vi "Slice Engine.vi"(7 "Table Stages":T3={"X Stage"={"Position"=0.0, "Is.Enabled?"=FALSE, "Is.Connected?"=FALSE, "Device SN"="45876425", "AccelerationMaximum"=20.0, "VelocityMaximum"=20.0, "Acceleration"=15.0, "Velocity"=18.0, "waitTimeout (ms)"=500000, "Model"=enum."None", "Is.Homed?"=FALSE, "MOVE"=FALSE}, "Y Stage"={"Position"=0.0, "Is.Enabled?"=FALSE, "Is.Connected?"=FALSE, "Device SN"="45995820", "AccelerationMaximum"=20.0, "VelocityMaximum"=20.0, "Acceleration"=15.0, "Velocity"=18.0, "waitTimeout (ms)"=5000000, "Model"=enum."None", "Is.Homed?"=FALSE, "MOVE"=FALSE}, "Z Stage"={"Position"=0.0, "Is.Enabled?"=FALSE, "Is.Connected?"=FALSE, "Device SN"="49103464", "AccelerationMaximum"=0.0, "VelocityMaximum"=0.0, "Acceleration"=0.0, "Velocity"=0.0, "waitTimeout (ms)"=0, "Model"=enum."None", "Is.Homed?"=FALSE, "MOVE"=FALSE}}, 8 "error in (no error)":errorcluster, 9 "Vibratome":T1={"Z Bottom [mm]"=0.0, "Pre Cut Dwell [s]"=0.0, "Blade Frequency [RPM]"=0, "Slice Speed [mm/s]"=0.0, "Post Cut Dwell [s]"=0.0, "Ramp Time [s]"=0.0, "Start X [mm]"=0.0, "Start Y [mm]"=0.0, "Slice Length [mm]"=0.0, "Slice Axis"=enum."X Axis", "Controller VISA Ref"="COM4", "Blade Frequency [Hz]"=0, "Analog Out Channel"="GalvoCtrl/ao0,GalvoCtrl/ao1", "Pixel Clock Source"="/GalvoCtrl/PFI0", "Vib"=enum."Vibratome1"}, 10 "Action":string="Init", 11 "Last Slice?":bool) -> (0 "error out":errorcluster)   [LabVIEW 2018]
uses:
  Controls/Translation Stage Parameters.ctl
  Hardware Mfg/Thorlabs Translation Stages/Controls/Translation Stage Cluster.ctl
  Controls/Translation Stage Types.ctl
  Controls/Vibratome Parameters.ctl
  type defines/vibratome.ctl
  Controls/Queue Manager Actions.ctl
  Controls/QueueNames.ctl
  Controls/Set Get Controls.ctl
  Hardware Mfg/Thorlabs Translation Stages/Controls/Motion Translation Module Control2.ctl
  Hardware Mfg/Thorlabs Translation Stages/Controls/Motion Translation Module Control.ctl
  Controls/vibratome3 control.ctl
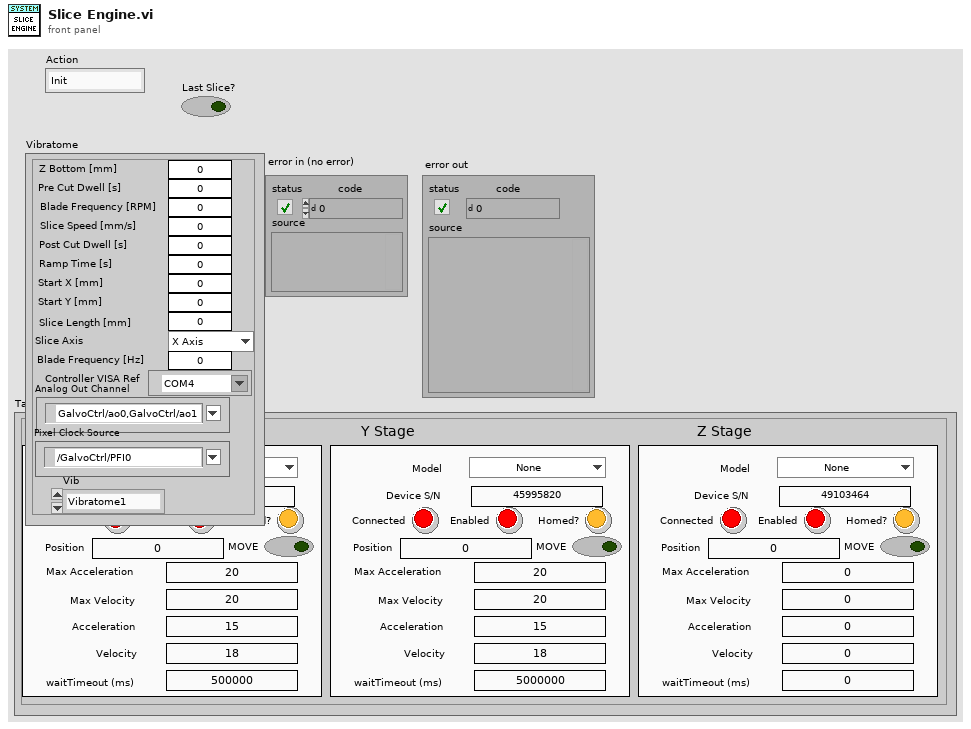
[diagram p1: front panel]
types:
  T1 = typedef "Vibratome Parameters.ctl" = cluster{"Z Bottom [mm]":dbl, "Pre Cut Dwell [s]":dbl, "Blade Frequency [RPM]":u16, "Slice Speed [mm/s]":dbl, "Post Cut Dwell [s]":dbl, "Ramp Time [s]":dbl, "Start X [mm]":dbl, "Start Y [mm]":dbl, "Slice Length [mm]":dbl, "Slice Axis":enum16{"X Axis", "Y Axis", "Z Axis"}, "Controller VISA Ref":refnum<visa-resource-name>, "Blade Frequency [Hz]":u16, "Analog Out Channel":tag, "Pixel Clock Source":tag, "Vib":T2}
  T2 = typedef "vibratome.ctl" = enum16{"Vibratome1", "Vibratome3"}
  T3 = typedef "Translation Stage Parameters.ctl" = cluster{"X Stage":T4, "Y Stage":T4, "Z Stage":T4}
  T4 = typedef "Translation Stage Cluster.ctl" = cluster{"Position":dbl, "Is.Enabled?":bool, "Is.Connected?":bool, "Device SN":string, "AccelerationMaximum":dbl, "VelocityMaximum":dbl, "Acceleration":dbl, "Velocity":dbl, "waitTimeout (ms)":i32, "Model":T5, "Is.Homed?":bool, "MOVE":bool}
  T5 = typedef "Translation Stage Types.ctl" = enum16{"None", "Thorlabs LTS", "Thorlabs MLJ"}
  T6 = typedef "QueueNames.ctl" = enum16{"Main GUI", "Main Scan Processor", "Main Processing", "Main Saving", "Main Display", "Main Table Stage GUI", "Main Table Stage Proc.", "Scan Engine", "Vibratome GUI", "Vibratome Processor", "Slice Engine"}
  T7 = typedef "Queue Manager Actions.ctl" = enum16{"Init", "Enqueue", "Enqueue All", "Preview Queue", "Dequeue", "Get Status", "Flush Queue", "Flush All Queues", "Release All Queues", "Release Queue", "Enqueue at Opposite End"}
  T8 = typedef "Set Get Controls.ctl" = enum16{"Set", "Get"}
  T9 = typedef "Motion Translation Module Control.ctl" = enum16{"Init", "Home", "Status", "Velocity/Accel", "Position", "Jog", "Stop", "Uninit", "Enable", "Disable"}
  T10 = typedef "Motion Translation Module Control2.ctl" = enum16{"Init", "Home", "Status", "Velocity/Accel", "Position", "Jog", "Stop", "Uninit", "Enable", "Disable"}
  T11 = enum16{"Set Configuration", "Get Configuration", "Enable Motor", "Disable Motor", "Get Status", "Open Session", "Close Session", "Set Limits", "Get Limits"}
  T12 = cluster{"Source for Velocity":enum16{"Interface", "Voltage (AI)", "PWM (AI)", "Current Target (AI)", "Current Target w/ Preset (AI)"}, "Mode":enum16{"Continuous", "Stepper Motor", "Analog Position Ctrl", "Encoder"}, "Target Velocity [RPM]":i16}
  T13 = typedef "vibratome3 control.ctl" = enum16{"Init", "Configure channel", "Write waveform", "Start", "Stop", "Finish?", "Uninit"}
  T14 = typedef "Motion Translation Module Control.ctl" = enum16{"Uninit", "Measure power", "Move angle", "Gen angles", "Init cage", "Init PM"}
  T15 = typedef "MessagePacket.ctl" = cluster{"Message":string, "Parameter":variant}
  T16 = typedef "Translation Stage Quick Status.ctl" = cluster{"Is.Enabled?":bool, "Is.Connected?":bool, "Is.Homed?":bool}
  T17 = enum16{"Left Button", "Center Button", "Right Button", "Window Close"}
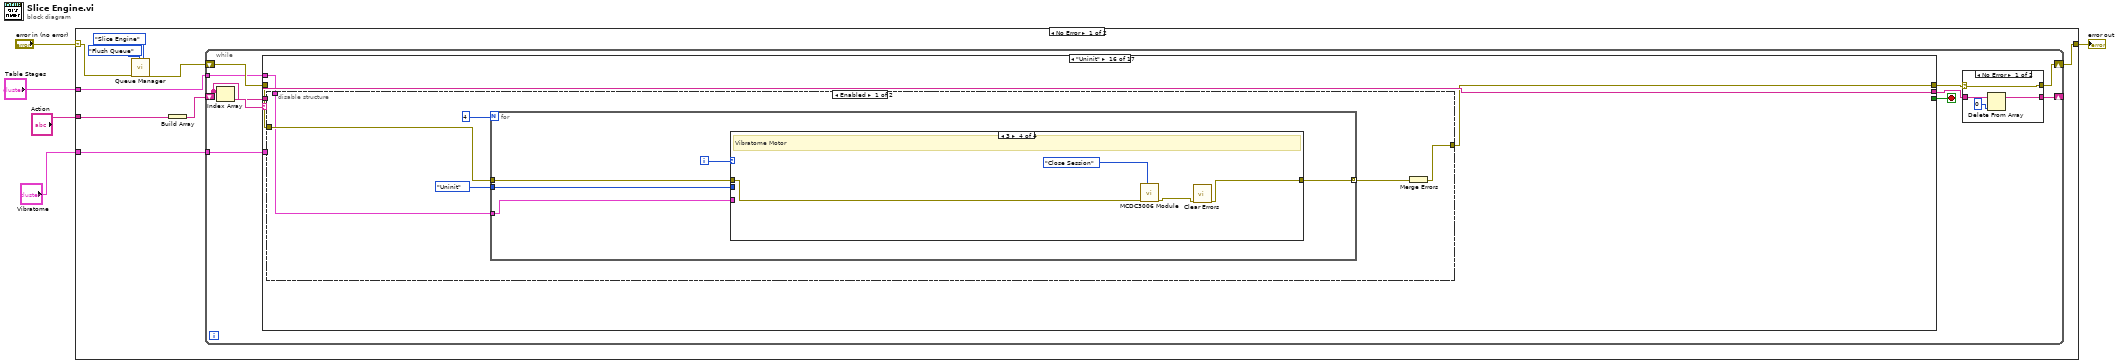
[diagram p0: block diagram]
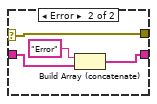
[diagram p2: hidden frame]
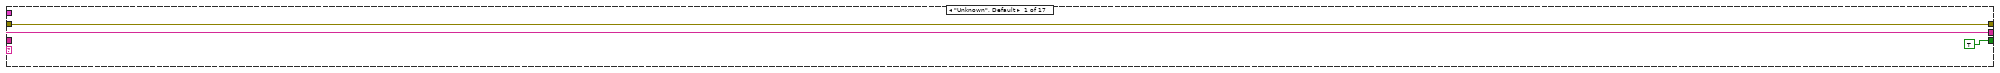
[diagram p3: hidden frame]
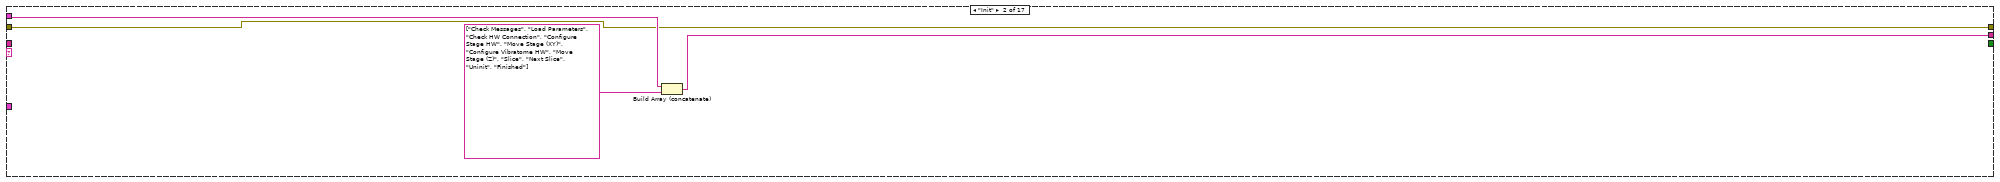
[diagram p4: hidden frame]
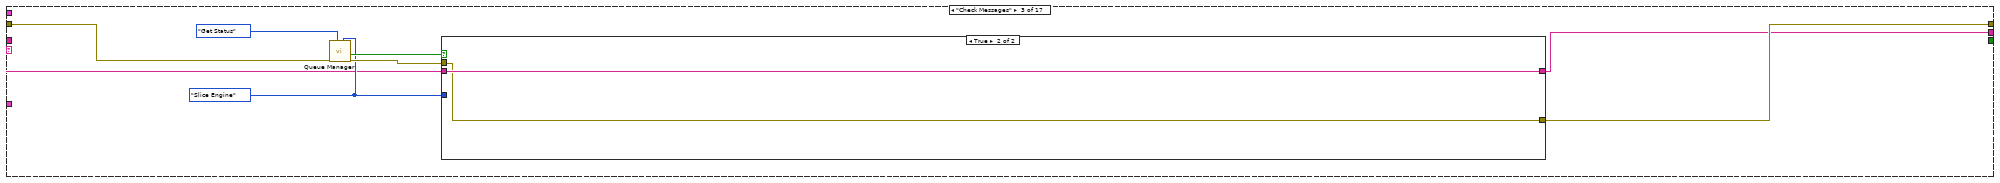
[diagram p5: hidden frame]
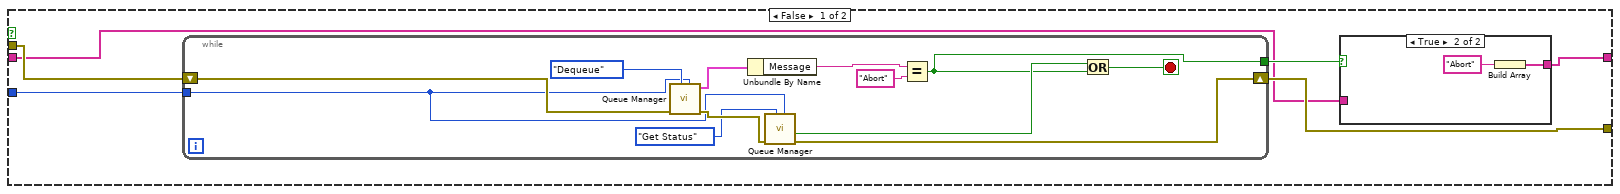
[diagram p6: hidden frame]
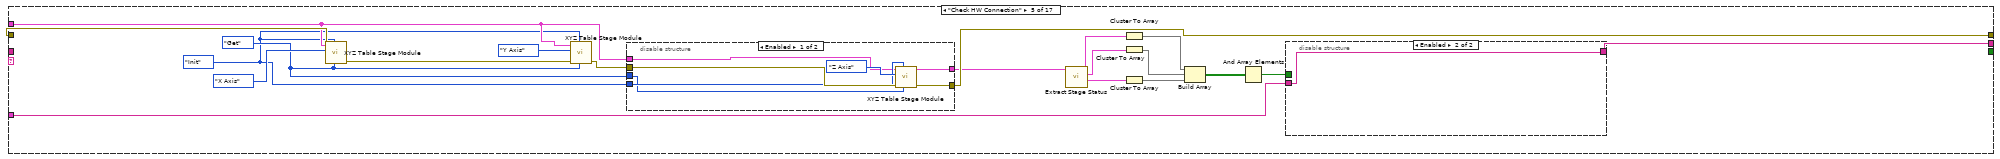
[diagram p9: hidden frame]
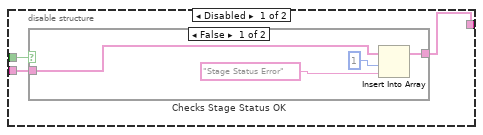
[diagram p10: hidden frame]
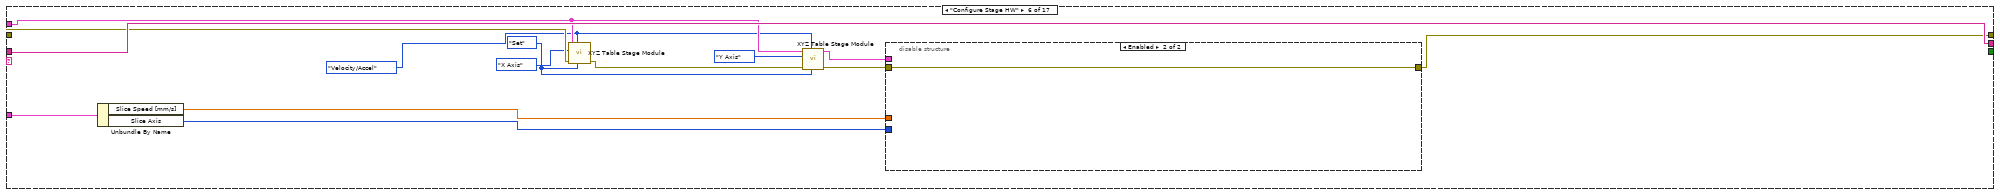
[diagram p13: hidden frame]
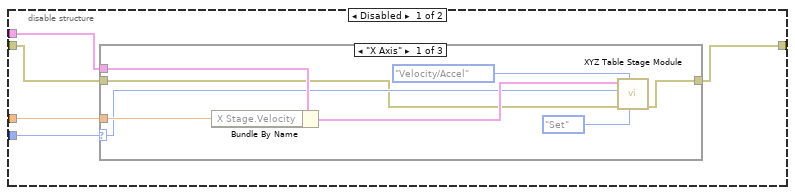
[diagram p14: hidden frame]
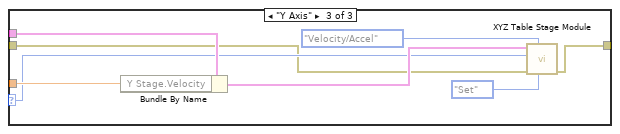
[diagram p16: hidden frame]
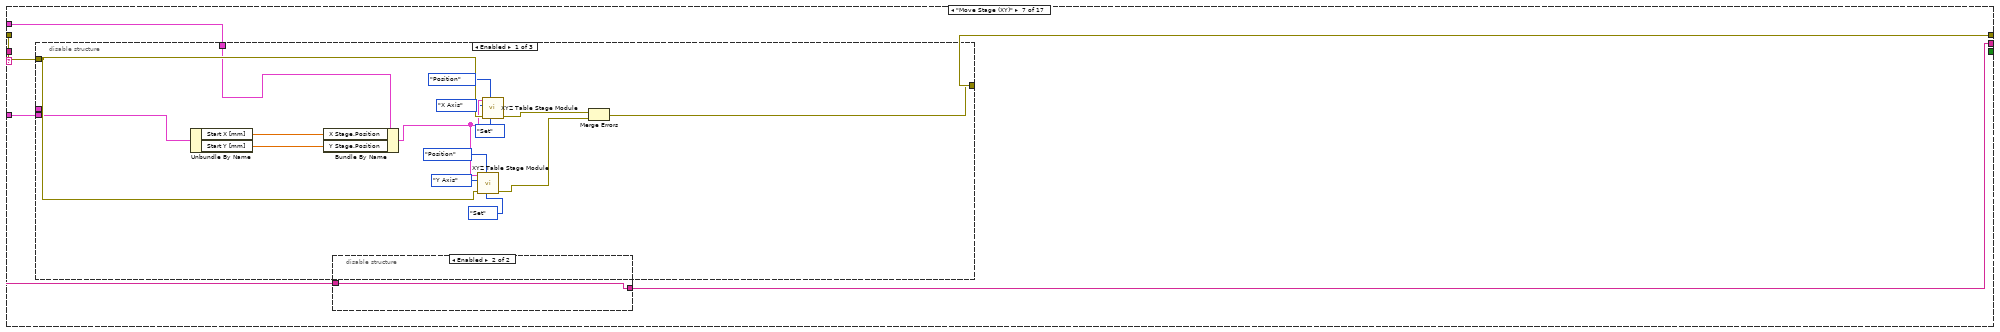
[diagram p17: hidden frame]
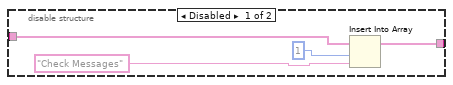
[diagram p18: hidden frame]
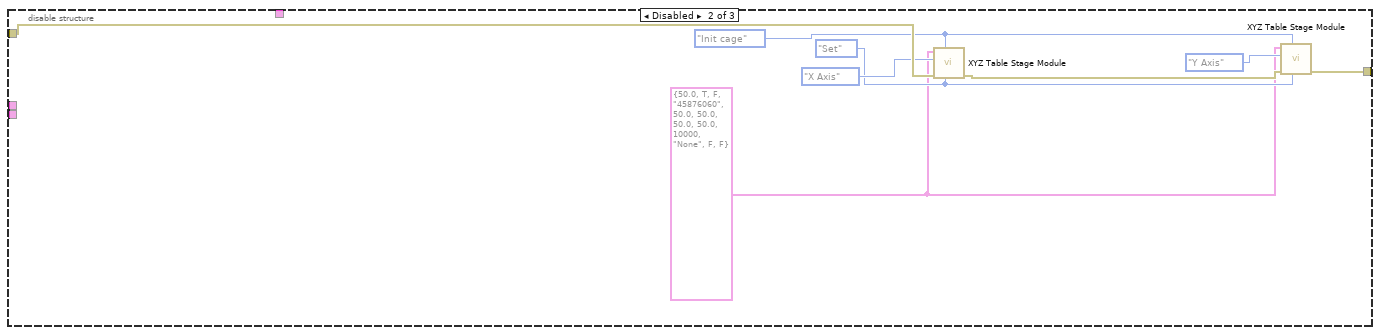
[diagram p19: hidden frame]
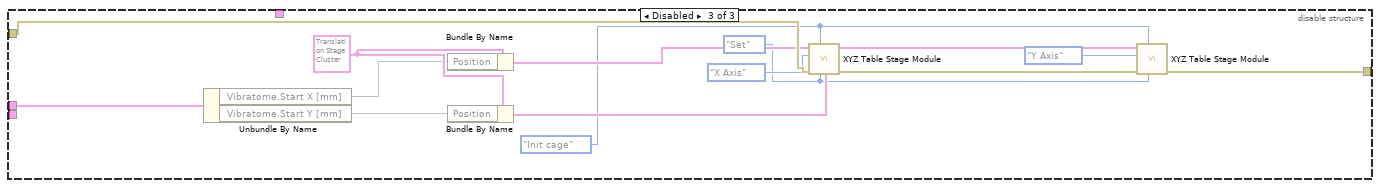
[diagram p20: hidden frame]
diagram:
  n1 = case shown="No Error" "error in (no error)" {
    selector: "error in (no error)" -> [w10 w528]
    tunnel: [w11 w528] -> w4
    tunnel: "Action" -> [w9 _]
    tunnel: "Table Stages" -> [w7 _]
    tunnel: "Vibratome" -> [w6 _]
    frame No Error {
      n2 = call "Queue Manager.vi"("Queue Name"=QueueNames."Slice Engine", "Action"=Queue_Manager_Actions."Flush Queue", "Error In"=w10) -> ("Error Out"=w8:errorcluster)  [unwired: 4 in, 4 out]
      n3 = Build Array(w9) -> (w12:string[])
      n4 = while {
        shift-right: [w19] -> _
        shift-left: w12 -> [w18]
        shift-right: [w21] -> w11
        shift-left: w8 -> [w24]
        tunnel: w7 -> [w17]
        tunnel: w6 -> [w16]
        stop <- w15 stop-if-true
        n5 = Index Array(array=w18) -> (element=w23:string)  [unwired: 1 in]
        n6 = case shown="\"Uninit\"" w23 {
          tunnel: w24 -> [w34 w36 w47 w71 w92 w123 w151 w201 w205 w213 w321 w364 w382 w406 w410 w439 w526]
          tunnel: w18 -> [w35 w39 w41 w72 w76 w124 w153 w202 w204 w216 w324 w367 w379 w403 w408 w440 w527]
          tunnel: [w35 w38 w40 w72 w77 w124 w152 w202 w203 w215 w323 w366 w379 w404 w407 w440 w527] -> w20
          tunnel: [w34 w36 w42 w71 w91 w114 w150 w195 w205 w214 w322 w364 w380 w406 w411 w438 w525] -> w22
          tunnel: w17 -> [_ _ _ _ w74 w113 w149 _ _ w211 w319 _ w378 _ _ w437 _]
          tunnel: w16 -> [_ _ _ _ _ w112 w148 w197 _ w212 w320 _ w377 _ _ _ _]
          tunnel: [TRUE _ _ _ _ _ _ _ _ _ _ _ _ _ _ _ TRUE] -> w15
          frame "Unknown", Default {
          }
          frame "Init" {
            n7 = Build Array (concatenate)(w39, string[] ["Check Messages", "Load Parameters", "Check HW Connection", "Configure Stage HW", "Move Stage (XY)", "Configure Vibratome HW", "Move Stage (Z)", "Slice", "Next Slice", "Uninit", "Finished"]) -> (w38:string[])
          }
          frame "Check Messages" {
            w43 = QueueNames."Slice Engine" ("Queue Name")
            n8 = call "Queue Manager.vi"("Queue Name"=w43, "Action"=Queue_Manager_Actions."Get Status", "Error In"=w47) -> ("Error Out"=w44:errorcluster, "Empty?"=w45:bool)  [unwired: 4 in, 3 out]
            n9 = case shown="True" w45 {
              tunnel: w44 -> [w53 w69]
              tunnel: w43 -> [w52 _]
              tunnel: [w51 w69] -> w42
              tunnel: w41 -> [w49 w70]
              tunnel: [w48 w70] -> w40
              frame False {
                n10 = while {
                  tunnel: w52 -> [w64]
                  shift-right: [w65] -> w51
                  shift-left: w53 -> [w68]
                  tunnel: [w57] -> w50
                  stop <- w58 stop-if-true
                  n11 = call "Queue Manager.vi"("Queue Name"=w64, "Action"=Queue_Manager_Actions."Dequeue", "Error In"=w68) -> ("Error Out"=w66:errorcluster, "Message Packet [Out]"=w62:T15)  [unwired: 4 in, 3 out]
                  n12 = Unbundle By Name(w62) -> ("Message"=w61:string)
                  n13 = call "Queue Manager.vi"("Queue Name"=w64, "Action"=Queue_Manager_Actions."Get Status", "Error In"=w66) -> ("Error Out"=w65:errorcluster, "Empty?"=w59:bool)  [unwired: 4 in, 3 out]
                  n14 = Equal?(x=w61, y="Abort") -> (x = y?=w57:bool)
                  n15 = Or(x=w59, y=w57) -> (x .or. y?=w58:bool)
                }
                n16 = case shown="True" w50 {
                  tunnel: w49 -> [w54 _]
                  tunnel: [w54 w55] -> w48
                  frame False {
                  }
                  frame True {
                    n17 = Build Array("Abort") -> (w55:string[])
                  }
                }
              }
              frame True {
              }
            }
          }
          frame "Load Parameters" {
          }
          frame "Check HW Connection" {
            w73 = Motion_Translation_Module_Control2."Init" ("Action")
            w86 = Set_Get_Controls."Get" ("Set/Get")
            n18 = call "XYZ Table Stage Module.vi"("Set/Get"=w86, "Action"=w73, "Error In"=w92, "Axis"=enum16{"X Axis", "Y Axis", "Z Axis"}."X Axis", "Table Stages"=w74) -> ("Error Out"=w90:errorcluster)  [unwired: 5 in, 1 out]
            n19 = call "XYZ Table Stage Module.vi"("Set/Get"=w86, "Action"=w73, "Error In"=w90, "Axis"=enum16{"X Axis", "Y Axis", "Z Axis"}."Y Axis", "Table Stages"=w74) -> ("Error Out"=w89:errorcluster)  [unwired: 5 in, 1 out]
            n20 = disable-structure shown="Enabled" {
              disable-tunnel: [w108 w110] -> w91
              disable-tunnel: w89 -> [w107 w110]
              disable-tunnel: w73 -> [w105 _]
              disable-tunnel: w86 -> [w104 _]
              disable-tunnel: w74 -> [w103 w109]
              disable-tunnel: [w102 w109] -> w85
              frame Enabled {
                n21 = call "XYZ Table Stage Module.vi"("Set/Get"=w104, "Action"=w105, "Error In"=w107, "Axis"=enum16{"X Axis", "Y Axis", "Z Axis"}."Z Axis", "Table Stages"=w103) -> ("Error Out"=w108:errorcluster, "Table Stages [out]"=w102:T3)  [unwired: 5 in]
              }
              frame Disabled {
              }
            }
            n22 = call "Extract Stage Status.vi"("Table Stages"=w85) -> ("Z Stage"=w82:T16, "Y Stage"=w83:T16, "X Stage"=w84:T16)  [unwired: 8 in]
            n23 = Cluster To Array(cluster=w84) -> (array=w81:bool[])
            n24 = Cluster To Array(cluster=w83) -> (array=w80:bool[])
            n25 = Cluster To Array(cluster=w82) -> (array=w79:bool[])
            n26 = Build Array(w81, w80, w79) -> (w78:bool[][])
            n27 = And Array Elements(Boolean array=w78) -> (logical AND=w75:bool)
            n28 = disable-structure shown="Enabled" {
              disable-tunnel: [w95 w101] -> w77
              disable-tunnel: w76 -> [w94 w101]
              disable-tunnel: w75 -> [w93 _]
              frame Disabled {
                n29 = case "Checks Stage Status OK" shown="False" w93 {
                  tunnel: [w99 w100] -> w95
                  tunnel: w94 -> [w98 w100]
                  frame False {
                    n30 = Insert Into Array(array=w98, index=1, new element="Stage Status Error" ("new element/subarray")) -> (w99:string[])
                  }
                  frame True {
                  }
                }
              }
              frame Enabled {
              }
            }
          }
          frame "Configure Stage HW" {
            w111 = Motion_Translation_Module_Control2."Velocity/Accel" ("Action")
            w119 = Set_Get_Controls."Set" ("Set/Get")
            n31 = Unbundle By Name(w112) -> ("Slice Speed [mm/s]"=w117:dbl, "Slice Axis"=w118:enum16{"X Axis", "Y Axis", "Z Axis"})
            n32 = call "XYZ Table Stage Module.vi"("Set/Get"=w119, "Action"=w111, "Error In"=w123, "Axis"=enum16{"X Axis", "Y Axis", "Z Axis"}."X Axis", "Table Stages"=w113) -> ("Error Out"=w122:errorcluster)  [unwired: 5 in, 1 out]
            n33 = call "XYZ Table Stage Module.vi"("Set/Get"=w119, "Action"=w111, "Error In"=w122, "Axis"=enum16{"X Axis", "Y Axis", "Z Axis"}."Y Axis", "Table Stages"=w113) -> ("Error Out"=w115:errorcluster, "Table Stages [out]"=w116:T3)  [unwired: 5 in]
            n34 = disable-structure shown="Enabled" {
              disable-tunnel: w118 -> [w129 _]
              disable-tunnel: w117 -> [w128 _]
              disable-tunnel: w116 -> [w127 _]
              disable-tunnel: w115 -> [w126 w147]
              disable-tunnel: [w125 w147] -> w114
              frame Disabled {
                n35 = case shown="\"X Axis\"" w129 {
                  selector: w129 -> [w134 _ w143]
                  tunnel: w128 -> [w137 _ w146]
                  tunnel: w127 -> [w136 _ w145]
                  tunnel: w126 -> [w133 w138 w142]
                  tunnel: [w132 w138 w141] -> w125
                  frame "X Axis" {
                    n36 = Bundle By Name(cluster=w136, "X Stage.Velocity"=w137) -> (w135:T3)
                    n37 = call "XYZ Table Stage Module.vi"("Set/Get"=Set_Get_Controls."Set", "Action"=Motion_Translation_Module_Control."Velocity/Accel", "Error In"=w133, "Axis"=w134, "Table Stages"=w135) -> ("Error Out"=w132:errorcluster)  [unwired: 5 in, 1 out]
                  }
                  frame "Z Axis" {
                  }
                  frame "Y Axis" {
                    n38 = Bundle By Name(cluster=w145, "Y Stage.Velocity"=w146) -> (w144:T3)
                    n39 = call "XYZ Table Stage Module.vi"("Set/Get"=Set_Get_Controls."Set", "Action"=Motion_Translation_Module_Control."Velocity/Accel", "Error In"=w142, "Axis"=w143, "Table Stages"=w144) -> ("Error Out"=w141:errorcluster)  [unwired: 5 in, 1 out]
                  }
                }
              }
              frame Enabled {
              }
            }
          }
          frame "Move Stage (XY)" {
            n40 = disable-structure shown="Enabled" {
              disable-tunnel: w151 -> [w169 w179 w192]
              disable-tunnel: [w173 w180 w193] -> w150
              disable-tunnel: _ -> [_ _ w191]
              disable-tunnel: w149 -> [w162 _ _]
              disable-tunnel: w148 -> [w161 _ _]
              frame Enabled {
                n41 = Unbundle By Name(w161) -> ("Start X [mm]"=w172:dbl, "Start Y [mm]"=w168:dbl)
                n42 = Bundle By Name(cluster=w162, "X Stage.Position"=w172, "Y Stage.Position"=w168) -> (w167:T3)
                n43 = call "XYZ Table Stage Module.vi"("Set/Get"=Set_Get_Controls."Set", "Action"=Motion_Translation_Module_Control2."Position", "Error In"=w169, "Axis"=enum16{"X Axis", "Y Axis", "Z Axis"}."Y Axis", "Table Stages"=w167) -> ("Error Out"=w171:errorcluster)  [unwired: 5 in, 1 out]
                n44 = call "XYZ Table Stage Module.vi"("Set/Get"=Set_Get_Controls."Set", "Action"=Motion_Translation_Module_Control2."Position", "Error In"=w169, "Axis"=enum16{"X Axis", "Y Axis", "Z Axis"}."X Axis", "Table Stages"=w167) -> ("Error Out"=w170:errorcluster)  [unwired: 5 in, 1 out]
                n45 = Merge Errors(w170, w171) -> (w173:errorcluster)
              }
              frame Disabled {
                w175 = Set_Get_Controls."Set" ("Set/Get")
                w176 = Motion_Translation_Module_Control."Init cage" ("Action")
                w174 = T4 {"Position"=50.0, "Is.Enabled?"=TRUE, "Is.Connected?"=FALSE, "Device SN"="45876060", "AccelerationMaximum"=50.0, "VelocityMaximum"=50.0, "Acceleration"=50.0, "Velocity"=50.0, "waitTimeout (ms)"=10000, "Model"=enum."None", "Is.Homed?"=FALSE, "MOVE"=FALSE} ("Cluster In")
                n46 = call "XYZ Table Stage Module.vi"("Set/Get"=w175, "Action"=w176, "Error In"=w179, "Axis"=enum16{"X Axis", "Y Axis", "Z Axis"}."X Axis", "Table Stages"=w174) -> ("Error Out"=w181:errorcluster)  [unwired: 5 in, 1 out]
                n47 = call "XYZ Table Stage Module.vi"("Set/Get"=w175, "Action"=w176, "Error In"=w181, "Axis"=enum16{"X Axis", "Y Axis", "Z Axis"}."Y Axis", "Table Stages"=w174) -> ("Error Out"=w180:errorcluster)  [unwired: 5 in, 1 out]
              }
              frame Disabled {
                w182 = Set_Get_Controls."Set" ("Set/Get")
                w183 = Motion_Translation_Module_Control."Init cage" ("Action")
                w190 = T4 {"Position"=0.0, "Is.Enabled?"=TRUE, "Is.Connected?"=FALSE, "Device SN"="45876060", "AccelerationMaximum"=50.0, "VelocityMaximum"=50.0, "Acceleration"=50.0, "Velocity"=50.0, "waitTimeout (ms)"=10000, "Model"=enum."None", "Is.Homed?"=FALSE, "MOVE"=FALSE} ("Cluster In")
                n48 = Unbundle By Name(w191) -> ("Vibratome.Start X [mm]"=w189, "Vibratome.Start Y [mm]"=w188)
                n49 = Bundle By Name(cluster=w190, "Position"=w189) -> (w187:T4)
                n50 = Bundle By Name(cluster=w190, "Position"=w188) -> (w186:T4)
                n51 = call "XYZ Table Stage Module.vi"("Set/Get"=w182, "Action"=w183, "Error In"=w192, "Axis"=enum16{"X Axis", "Y Axis", "Z Axis"}."X Axis", "Table Stages"=w187) -> ("Error Out"=w194:errorcluster)  [unwired: 5 in, 1 out]
                n52 = call "XYZ Table Stage Module.vi"("Set/Get"=w182, "Action"=w183, "Error In"=w194, "Axis"=enum16{"X Axis", "Y Axis", "Z Axis"}."Y Axis", "Table Stages"=w186) -> ("Error Out"=w193:errorcluster)  [unwired: 5 in, 1 out]
              }
            }
            n53 = disable-structure shown="Enabled" {
              disable-tunnel: w153 -> [w157 w158]
              disable-tunnel: [w156 w158] -> w152
              frame Disabled {
                n54 = Insert Into Array(array=w157, index=1, new element="Check Messages" ("new element/subarray")) -> (w156:string[])
              }
              frame Enabled {
              }
            }
          }
          frame "Configure Vibratome HW" {
            n55 = Unbundle By Name(w197) -> ("Controller VISA Ref"=w196:refnum<visa-resource-name>)
            n56 = call "MCDC3006 Module.vi"("Actions"=T11."Open Session", "Error In"=w201, "VISA resource name"=w196) -> ("Error Out"=w198:errorcluster)  [unwired: 4 in, 4 out]
            n57 = call "MCDC3006 Module.vi"("Actions"=T11."Enable Motor", "Error In"=w198, "VISA resource name"=w196) -> ("Error Out"=w195:errorcluster)  [unwired: 4 in, 4 out]
          }
          frame "Move Stage (Z)" {
            n58 = disable-structure shown="Disabled" {
              disable-tunnel: w204 -> [w209 w210]
              disable-tunnel: [w208 w210] -> w203
              frame Disabled {
                n59 = Insert Into Array(array=w209, index=1, new element="Check Messages" ("new element/subarray")) -> (w208:string[])
              }
              frame Enabled {
              }
            }
          }
          frame "Slice" {
            n60 = disable-structure shown="Enabled" {
              disable-tunnel: _ -> [_ w292]
              disable-tunnel: [w226 w293] -> w214
              disable-tunnel: w213 -> [w241 w294]
              disable-tunnel: w212 -> [w238 _]
              disable-tunnel: w211 -> [w237 _]
              disable-tunnel: w211 -> [w225 _]
              frame Enabled {
                n61 = Unbundle By Name(w238) -> ("Controller VISA Ref"=w236:refnum<visa-resource-name>, "Blade Frequency [RPM]"=w247:u16, "Slice Axis"=w252:enum16{"X Axis", "Y Axis", "Z Axis"}, "Slice Length [mm]"=w251:dbl, "Post Cut Dwell [s]"=w245:dbl, "Pre Cut Dwell [s]"=w244:dbl, "Slice Speed [mm/s]"=w243:dbl, "Start X [mm]"=w239:dbl)
                n62 = Bundle By Name(cluster=T12 {"Source for Velocity"=enum."Interface", "Mode"=enum."Continuous", "Target Velocity [RPM]"=0} ("Configuration [In]"), "Target Velocity [RPM]"=w247) -> (w246:T12)
                n63 = call "MCDC3006 Module.vi"("Actions"=T11."Enable Motor", "Error In"=w241, "VISA resource name"=w236) -> ("Error Out"=w240:errorcluster)  [unwired: 4 in, 4 out]
                n64 = call "MCDC3006 Module.vi"("Actions"=T11."Set Configuration", "Error In"=w240, "Configuration [In]"=w246, "VISA resource name"=w236) -> ("Error Out"=w250:errorcluster)  [unwired: 3 in, 4 out]
                n65 = case shown="\"X Axis\"" w252 {
                  tunnel: w250 -> [w273 w274 w290]
                  tunnel: [w264 w274 w277] -> w227
                  tunnel: w251 -> [w267 _ w284]
                  tunnel: w245 -> [w262 _ w280]
                  tunnel: w244 -> [w270 _ _]
                  tunnel: w243 -> [_ _ _]
                  tunnel: w239 -> [w257 _ _]
                  tunnel: w237 -> [w254 _ _]
                  frame "X Axis" {
                    n66 = expression code="x*1000"(w270) -> (w269:dbl)
                    n67 = To Unsigned Long Integer(number=w269) -> (unsigned 32bit integer=w268:u32)
                    n68 = call "Inline Wait.vi"("Error In"=w273, "milliseconds to wait"=w268) -> ("Error Out"=w259:errorcluster)  [unwired: 9 in]
                    n69 = Multiply(x=w262, y=1000.0) -> (x*y=w265:dbl)
                    n70 = Subtract(x=w257, y=w267) -> (x-y=w272:dbl)
                    n71 = To Unsigned Long Integer(number=w265) -> (unsigned 32bit integer=w271:u32)
                    n72 = Bundle By Name(cluster=w254, "X Stage.Position"=w272) -> (w256:T3)
                    n73 = call "XYZ Table Stage Module.vi"("Set/Get"=Set_Get_Controls."Set", "Action"=Motion_Translation_Module_Control2."Position", "Error In"=w259, "Axis"=enum16{"X Axis", "Y Axis", "Z Axis"}."X Axis", "Table Stages"=w256) -> ("Error Out"=w258:errorcluster)  [unwired: 5 in, 1 out]
                    n74 = call "Inline Wait.vi"("Error In"=w258, "milliseconds to wait"=w271) -> ("Error Out"=w255:errorcluster)  [unwired: 9 in]
                    n75 = call "MCDC3006 Module.vi"("Actions"=T11."Disable Motor", "Error In"=w255) -> ("Error Out"=w264:errorcluster)  [unwired: 5 in, 4 out]
                  }
                  frame "Z Axis" {
                  }
                  frame "Y Axis" {
                    (unwired) Motion_Translation_Module_Control."Init cage" ("Action")
                    n76 = expression code="x*1000"(w280) -> (w279:dbl)
                    n77 = call "Thorlabs LTS - Y Stage Module.vi"("Set/Get"=Set_Get_Controls."Get", "Error In"=w290) -> ("Error Out"=w289:errorcluster, "Cluster Out"=w275:T4)  [unwired: 8 in]
                    n78 = Unbundle By Name(w275) -> ("Position"=w285:dbl)
                    n79 = To Unsigned Long Integer(number=w279) -> (unsigned 32bit integer=w278:u32)
                    n80 = Add(x=w285, y=w284) -> (x+y=w283:dbl)
                    n81 = Bundle By Name(cluster=w275, "Position"=w283) -> (w282:T4)
                    n82 = call "Thorlabs LTS - Y Stage Module.vi"("Set/Get"=Set_Get_Controls."Set", "Error In"=w289, "Cluster In"=w282) -> ("Error Out"=w287:errorcluster)  [unwired: 7 in, 1 out]
                    n83 = call "Inline Wait.vi"("Error In"=w287, "milliseconds to wait"=w278) -> ("Error Out"=w281:errorcluster)  [unwired: 9 in]
                    n84 = call "Thorlabs LTS - Y Stage Module.vi"("Set/Get"=Set_Get_Controls."Set", "Error In"=w281, "Cluster In"=w275) -> ("Error Out"=w277:errorcluster)  [unwired: 7 in, 1 out]
                  }
                }
                n85 = call "XYZ Table Stage Module.vi"("Set/Get"=Set_Get_Controls."Set", "Action"=Motion_Translation_Module_Control2."Velocity/Accel", "Error In"=w227, "Axis"=enum16{"X Axis", "Y Axis", "Z Axis"}."X Axis", "Table Stages"=w225) -> ("Error Out"=w235:errorcluster)  [unwired: 5 in, 1 out]
                n86 = call "XYZ Table Stage Module.vi"("Set/Get"=Set_Get_Controls."Set", "Action"=Motion_Translation_Module_Control2."Velocity/Accel", "Error In"=w235, "Axis"=enum16{"X Axis", "Y Axis", "Z Axis"}."Y Axis", "Table Stages"=w225) -> ("Error Out"=w230:errorcluster)  [unwired: 5 in, 1 out]
                n87 = call "XYZ Table Stage Module.vi"("Set/Get"=Set_Get_Controls."Set", "Action"=Motion_Translation_Module_Control2."Velocity/Accel", "Error In"=w230, "Axis"=enum16{"X Axis", "Y Axis", "Z Axis"}."Z Axis", "Table Stages"=w225) -> ("Error Out"=w226:errorcluster)  [unwired: 5 in, 1 out]
              }
              frame Disabled {
                n88 = Unbundle By Name(w292) -> ("Vibratome"=w291)
                n89 = call "Slice Module.vi"("Error In"=w294, "Vibratome"=w291) -> ("Error Out"=w293:errorcluster)  [unwired: 7 in, 2 out]
              }
            }
            n90 = disable-structure shown="Enabled" {
              disable-tunnel: w216 -> [w220 w221]
              disable-tunnel: [w219 w221] -> w215
              frame Disabled {
                n91 = Insert Into Array(array=w220, index=1, new element="Check Messages" ("new element/subarray")) -> (w219:string[])
              }
              frame Enabled {
              }
            }
          }
          frame "Slice3" {
            n92 = disable-structure shown="Enabled" {
              disable-tunnel: w324 -> [w362 w363]
              disable-tunnel: [w361 w363] -> w323
              frame Disabled {
                n93 = Insert Into Array(array=w362, index=1, new element="Check Messages" ("new element/subarray")) -> (w361:string[])
              }
              frame Enabled {
              }
            }
            n94 = Unbundle By Name(w320) -> ("Slice Axis"=w317:enum16{"X Axis", "Y Axis", "Z Axis"}, "Slice Length [mm]"=w316:dbl, "Ramp Time [s]"=w296:dbl, "Slice Speed [mm/s]"=w315:dbl, "Start X [mm]"=w314:dbl, "Start Y [mm]"=w295:dbl)  [unwired: 1 out]
            n95 = flat-sequence {
              tunnel: w321 -> [w333]
              tunnel: [w325] -> w318
              tunnel: [w337] -> w302
              tunnel: w318 -> [w337]
              tunnel: w296 -> [w334]
              frame #0 {
                n96 = call "vibratome3 module.vi"("Action"=vibratome3_control."Init", "error in"=w333) -> ("error out"=w328:errorcluster)  [unwired: 9 in]
                n97 = call "vibratome3 module.vi"("Action"=vibratome3_control."Configure channel", "error in"=w328) -> ("error out"=w327:errorcluster)  [unwired: 9 in]
                n98 = call "vibratome3 module.vi"("Action"=vibratome3_control."Write waveform", "error in"=w327) -> ("error out"=w326:errorcluster)  [unwired: 9 in]
                n99 = call "vibratome3 module.vi"("Action"=vibratome3_control."Start", "error in"=w326) -> ("error out"=w325:errorcluster)  [unwired: 9 in]
              }
              frame #1 {
                n100 = Multiply(x=w334, y=1000.0) -> (x*y=w336:dbl)
                n101 = Wait (ms)(milliseconds to wait=w336) -> ()  [unwired: 1 out]
              }
            }
            n102 = case shown="\"Y Axis\"" w317 {
              tunnel: w302 -> [w338 w349 w358]
              tunnel: [w339 w350 w358] -> w298
              tunnel: w316 -> [w346 w356 _]
              tunnel: w315 -> [_ _ _]
              tunnel: w314 -> [w343 _ _]
              tunnel: w319 -> [w341 w352 _]
              tunnel: w295 -> [_ w348 _]
              frame "X Axis", Default {
                n103 = Subtract(x=w343, y=w346) -> (x-y=w347:dbl)
                n104 = Bundle By Name(cluster=w341, "X Stage.Position"=w347) -> (w342:T3)
                n105 = call "XYZ Table Stage Module.vi"("Set/Get"=Set_Get_Controls."Set", "Action"=Motion_Translation_Module_Control2."Position", "Error In"=w338, "Axis"=enum16{"X Axis", "Y Axis", "Z Axis"}."X Axis", "Table Stages"=w342) -> ("Error Out"=w339:errorcluster)  [unwired: 5 in, 1 out]
              }
              frame "Y Axis" {
                n106 = Subtract(x=w348, y=w356) -> (x-y=w357:dbl)
                n107 = Bundle By Name(cluster=w352, "Y Stage.Position"=w357) -> (w353:T3)
                n108 = call "XYZ Table Stage Module.vi"("Set/Get"=Set_Get_Controls."Set", "Action"=Motion_Translation_Module_Control2."Position", "Error In"=w349, "Axis"=enum16{"X Axis", "Y Axis", "Z Axis"}."Y Axis", "Table Stages"=w353) -> ("Error Out"=w350:errorcluster)  [unwired: 5 in, 1 out]
              }
              frame "Z Axis" {
              }
            }
            n109 = call "vibratome3 module.vi"("Action"=vibratome3_control."Finish?", "error in"=w298) -> ("error out"=w299:errorcluster)  [unwired: 9 in]
            n110 = call "vibratome3 module.vi"("Action"=vibratome3_control."Uninit", "error in"=w299) -> ("error out"=w297:errorcluster)  [unwired: 9 in]
            n111 = call "XYZ Table Stage Module.vi"("Set/Get"=Set_Get_Controls."Set", "Action"=Motion_Translation_Module_Control2."Velocity/Accel", "Error In"=w297, "Axis"=enum16{"X Axis", "Y Axis", "Z Axis"}."X Axis", "Table Stages"=w319) -> ("Error Out"=w313:errorcluster)  [unwired: 5 in, 1 out]
            n112 = call "XYZ Table Stage Module.vi"("Set/Get"=Set_Get_Controls."Set", "Action"=Motion_Translation_Module_Control2."Velocity/Accel", "Error In"=w313, "Axis"=enum16{"X Axis", "Y Axis", "Z Axis"}."Y Axis", "Table Stages"=w319) -> ("Error Out"=w308:errorcluster)  [unwired: 5 in, 1 out]
            n113 = call "XYZ Table Stage Module.vi"("Set/Get"=Set_Get_Controls."Set", "Action"=Motion_Translation_Module_Control2."Velocity/Accel", "Error In"=w308, "Axis"=enum16{"X Axis", "Y Axis", "Z Axis"}."Z Axis", "Table Stages"=w319) -> ("Error Out"=w322:errorcluster)  [unwired: 5 in, 1 out]
          }
          frame "Next Slice" {
            n114 = case shown="True" "Last Slice?" {
              tunnel: w367 -> [w371 w373]
              tunnel: [w370 w372] -> w366
              frame False {
                n115 = Insert Into Array(array=w371, index=1, new element=string[] ["Move Stage (Z)", "Slice", "Next Slice"]) -> (w370:string[])
              }
              frame True {
                n116 = Insert Into Array(array=w373, index=1, new element=string[] ["Configure Stage HW", "", ""]) -> (w372:string[])
              }
            }
          }
          frame "Set Slice Speed" {
            n117 = Unbundle By Name(w377) -> ("Slice Axis"=w376:enum16{"X Axis", "Y Axis", "Z Axis"}, "Slice Speed [mm/s]"=w381:dbl)
            n118 = case shown="\"Y Axis\"" w376 {
              tunnel: w382 -> [w388 w398]
              tunnel: w381 -> [w387 w399]
              tunnel: [w386 w395] -> w380
              tunnel: w378 -> [w385 w394]
              frame "X Axis", Default {
                n119 = Bundle By Name(cluster=w385, "X Stage.Velocity"=w387, "X Stage.Acceleration"=50.0 ("Acceleration")) -> (w384:T3)
                n120 = call "XYZ Table Stage Module.vi"("Set/Get"=Set_Get_Controls."Set", "Action"=Motion_Translation_Module_Control2."Velocity/Accel", "Error In"=w388, "Axis"=enum16{"X Axis", "Y Axis", "Z Axis"}."X Axis", "Table Stages"=w384) -> ("Error Out"=w386:errorcluster)  [unwired: 5 in, 1 out]
              }
              frame "Y Axis" {
                n121 = Bundle By Name(cluster=w394, "Y Stage.Velocity"=w399, "Y Stage.Acceleration"=50.0 ("Acceleration")) -> (w393:T3)
                n122 = call "XYZ Table Stage Module.vi"("Set/Get"=Set_Get_Controls."Set", "Action"=Motion_Translation_Module_Control2."Velocity/Accel", "Error In"=w398, "Axis"=enum16{"X Axis", "Y Axis", "Z Axis"}."Y Axis", "Table Stages"=w393) -> ("Error Out"=w395:errorcluster)  [unwired: 5 in, 1 out]
              }
            }
          }
          frame "Abort" {
            n123 = Insert Into Array(array=w403, index=1, new element #1="Uninit", new element #2="Finished") -> (w404:string[])
          }
          frame "Error" {
            n124 = Unbundle(w410) -> ("code"=w420:i32, "source"=w419:string)  [unwired: 1 out]
            n125 = control-ref of="This VI"() -> (w421:refnum<vi>)
            n126 = property class="VI"(reference=w421) -> ("Name"=w424:string, "Callers"=w426:string[])  [unwired: 1 in, 2 out]
            n127 = Array To Spreadsheet String(delimiter (Tab)=">", array=w426, 3:"%s" ("format string")) -> (spreadsheet string=w425:string)
            n128 = Format Into String(format string="VI Name: %s\nCallers: %s\nError Code: %d\nError Message: %s", initial string="The following error occurred:\n" ("message"), w424, w425, w420, w419) -> (resulting string=w418:string, error out=w412:errorcluster)  [unwired: 1 in]
            n129 = call <vilib>:"Clear Errors.vi"("error in (no error)"=w412) -> ()  [unwired: 5 in, 2 out]
            n130 = call <vilib>:"Three Button Dialog.vi"("Allow user to close window? (TRUE)"=FALSE, "Window Title (\"\")"="Error" ("Window Title (\"\")"), "Right Button Text (\"Cancel\")"="Abort" ("Right Button Text (\"Cancel\")"), "Center Button Text (\"No\")"="Retry" ("Center Button Text (\"No\")"), "Left Button Text (\"Yes\")"="Continue" ("Left Button Text (\"Yes\")"), "message"=w418) -> ("Which Button?"=w409:T17)  [unwired: 5 in]
            n131 = case shown="\"Right Button\"" w409 {
              tunnel: w408 -> [w431 w435 w436]
              tunnel: [w430 w434 w436] -> w407
              frame "Left Button", Default {
                # "Continue"
                n132 = Delete From Array(array=w431, index=0) -> (array with subset deleted=w430:string[])  [unwired: 1 in, 1 out]
              }
              frame "Right Button" {
                # "Abort"
                n133 = Insert Into Array(array=w435, index=1, new element="Abort") -> (w434:string[])
              }
              frame "Center Button" {
                # "Retry"
              }
            }
            n134 = call <vilib>:"Clear Errors.vi"("error in (no error)"=w410) -> ("error out"=w411:errorcluster)  [unwired: 5 in, 1 out]
          }
          frame "Uninit" {
            n135 = disable-structure shown="Enabled" {
              disable-tunnel: w439 -> [w444 w522]
              disable-tunnel: [w443 w515] -> w438
              disable-tunnel: w437 -> [w441 _]
              frame Enabled {
                n136 = for {
                  N: 4 -> [_]
                  tunnel: [w450] -> w445 mode=indexing
                  tunnel: Motion_Translation_Module_Control."Uninit" ("Action") -> [w449]
                  tunnel: w444 -> [w448]
                  tunnel: w441 -> [w447]
                  i -> [w451]
                  n137 = case shown="3" w451 {
                    tunnel: [w455 w473 w491 w507] -> w450
                    tunnel: w448 -> [w454 w472 w490 w506]
                    tunnel: w449 -> [w453 w471 w489 _]
                    tunnel: w447 -> [w452 w470 w488 _]
                    frame 0, Default {
                      # "X Stage"
                      n138 = disable-structure shown="Enabled" {
                        disable-tunnel: [w461 _] -> w455
                        disable-tunnel: w454 -> [w460 _]
                        disable-tunnel: w453 -> [w459 _]
                        disable-tunnel: w452 -> [w456 _]
                        frame Disabled {
                          n139 = Unbundle By Name(w456) -> ("X Stage.Model"=w458:T5, "X Stage.Device SN"=w457:string)
                          n140 = case shown="\"Thorlabs LTS\"" w458 {
                            tunnel: [w462 w469] -> w461
                            tunnel: w460 -> [w462 w468]
                            tunnel: w459 -> [_ w467]
                            tunnel: w457 -> [_ w465]
                            frame "None", Default {
                            }
                            frame "Thorlabs LTS" {
                              n141 = Bundle By Name(cluster=T4 {"Position"=0.0, "Is.Enabled?"=TRUE, "Is.Connected?"=FALSE, "Device SN"="45876539", "AccelerationMaximum"=0.0, "VelocityMaximum"=0.0, "Acceleration"=0.0, "Velocity"=0.0, "waitTimeout (ms)"=0, "Model"=enum."Thorlabs LTS", "Is.Homed?"=FALSE, "MOVE"=FALSE} ("Cluster In"), "Device SN"=w465) -> (w464:T4)
                              n142 = call "Thorlabs LTS - X Stage Module.vi"("Set/Get"=Set_Get_Controls."Set", "Error In"=w468, "Action"=w467, "Cluster In"=w464) -> ("Error Out"=w469:errorcluster)  [unwired: 6 in, 1 out]
                            }
                          }
                        }
                        frame Enabled {
                        }
                      }
                    }
                    frame 1 {
                      # "Y Stage"
                      n143 = disable-structure shown="Enabled" {
                        disable-tunnel: [w479 _] -> w473
                        disable-tunnel: w472 -> [w478 _]
                        disable-tunnel: w471 -> [w477 _]
                        disable-tunnel: w470 -> [w474 _]
                        frame Disabled {
                          n144 = Unbundle By Name(w474) -> ("Y Stage.Model"=w476:T5, "Y Stage.Device SN"=w475:string)
                          n145 = case shown="\"Thorlabs LTS\"" w476 {
                            tunnel: [w480 w487] -> w479
                            tunnel: w478 -> [w480 w486]
                            tunnel: w477 -> [_ w485]
                            tunnel: w475 -> [_ w483]
                            frame "None", Default {
                            }
                            frame "Thorlabs LTS" {
                              n146 = Bundle By Name(cluster=T4 {"Position"=0.0, "Is.Enabled?"=TRUE, "Is.Connected?"=FALSE, "Device SN"="45876539", "AccelerationMaximum"=0.0, "VelocityMaximum"=0.0, "Acceleration"=0.0, "Velocity"=0.0, "waitTimeout (ms)"=0, "Model"=enum."Thorlabs LTS", "Is.Homed?"=FALSE, "MOVE"=FALSE} ("Cluster In"), "Device SN"=w483) -> (w482:T4)
                              n147 = call "Thorlabs LTS - Y Stage Module.vi"("Set/Get"=Set_Get_Controls."Set", "Error In"=w486, "Action"=w485, "Cluster In"=w482) -> ("Error Out"=w487:errorcluster)  [unwired: 6 in, 1 out]
                            }
                          }
                        }
                        frame Enabled {
                        }
                      }
                    }
                    frame 2 {
                      # "Z Stage"
                      n148 = disable-structure shown="Enabled" {
                        disable-tunnel: [w497 _] -> w491
                        disable-tunnel: w490 -> [w496 _]
                        disable-tunnel: w489 -> [w495 _]
                        disable-tunnel: w488 -> [w492 _]
                        frame Disabled {
                          n149 = Unbundle By Name(w492) -> ("Z Stage.Model"=w494:T5, "Z Stage.Device SN"=w493:string)
                          n150 = case shown="\"Thorlabs MLJ\"" w494 {
                            tunnel: [w498 w505] -> w497
                            tunnel: w496 -> [w498 w504]
                            tunnel: w495 -> [_ w503]
                            tunnel: w493 -> [_ w501]
                            frame "None", Default {
                            }
                            frame "Thorlabs MLJ" {
                              n151 = Bundle By Name(cluster=T4 {"Position"=0.0, "Is.Enabled?"=TRUE, "Is.Connected?"=FALSE, "Device SN"="45876539", "AccelerationMaximum"=0.0, "VelocityMaximum"=0.0, "Acceleration"=0.0, "Velocity"=0.0, "waitTimeout (ms)"=0, "Model"=enum."Thorlabs MLJ", "Is.Homed?"=FALSE, "MOVE"=FALSE} ("Cluster In"), "Device SN"=w501) -> (w500:T4)
                              n152 = call "Thorlabs MLJ - Z Stage Module.vi"("Set/Get"=Set_Get_Controls."Set", "Error In"=w504, "Action"=w503, "Cluster In"=w500) -> ("Error Out"=w505:errorcluster)  [unwired: 6 in, 1 out]
                            }
                          }
                        }
                        frame Enabled {
                        }
                      }
                    }
                    frame 3 {
                      # "Vibratome Motor"
                      n153 = call "MCDC3006 Module.vi"("Actions"=T11."Close Session", "Error In"=w506) -> ("Error Out"=w508:errorcluster)  [unwired: 5 in, 4 out]
                      n154 = call <vilib>:"Clear Errors.vi"("error in (no error)"=w508) -> ("error out"=w507:errorcluster)  [unwired: 5 in, 1 out]
                    }
                  }
                }
                n155 = Merge Errors(w445) -> (w443:errorcluster)
              }
              frame Disabled {
                w510 = Set_Get_Controls."Set" ("Set/Get")
                w514 = Motion_Translation_Module_Control."Uninit" ("Action")
                n156 = call "XYZ Table Stage Module.vi"("Set/Get"=w510, "Action"=w514, "Error In"=w522, "Axis"=enum16{"X Axis", "Y Axis", "Z Axis"}."X Axis") -> ("Error Out"=w521:errorcluster)  [unwired: 6 in, 1 out]
                n157 = call "XYZ Table Stage Module.vi"("Set/Get"=w510, "Action"=w514, "Error In"=w521, "Axis"=enum16{"X Axis", "Y Axis", "Z Axis"}."Y Axis") -> ("Error Out"=w520:errorcluster)  [unwired: 6 in, 1 out]
                n158 = call "XYZ Table Stage Module.vi"("Set/Get"=w510, "Action"=w514, "Error In"=w520, "Axis"=enum16{"X Axis", "Y Axis", "Z Axis"}."Z Axis") -> ("Error Out"=w517:errorcluster)  [unwired: 6 in, 1 out]
                n159 = call "MCDC3006 Module.vi"("Actions"=T11."Disable Motor", "Error In"=w517) -> ("Error Out"=w516:errorcluster)  [unwired: 5 in, 4 out]
                n160 = call "MCDC3006 Module.vi"("Actions"=T11."Close Session", "Error In"=w516) -> ("Error Out"=w515:errorcluster)  [unwired: 5 in, 4 out]
              }
            }
          }
          frame "Finished" {
            n161 = call "Inline Wait.vi"("Error In"=w526, "milliseconds to wait"=u32 1000) -> ("Error Out"=w525:errorcluster)  [unwired: 9 in]
          }
        }
        n162 = case shown="No Error" w22 {
          selector: w22 -> [w28 w29]
          tunnel: [w28 w29] -> w21
          tunnel: w20 -> [w27 w32]
          tunnel: [w26 w30] -> w19
          frame No Error {
            n163 = Delete From Array(array=w27, index=0) -> (array with subset deleted=w26:string[])  [unwired: 1 in, 1 out]
          }
          frame Error {
            n164 = Build Array (concatenate)("Error", w32) -> (w30:string[])
          }
        }
      }
    }
    frame Error {
    }
  }
  "error out" <- w4
